vi "Set Hover.vi"(8 "error in (no error)":errorcluster, 9 "Set Hover (F)":bool, 10 "Index":i32, 11 "MCListbox with Checkboxes in":refnum<class "MCListbox with Checkboxes.lvclass">) -> (0 "error out":errorcluster, 3 "MCListbox with Checkboxes out":refnum<class "MCListbox with Checkboxes.lvclass">)   [LabVIEW 2016, in "MCListbox with Checkboxes.lvclass"]
uses:
  MCListbox with Checkboxes.lvclass
  MCListbox with Checkboxes.lvclass/MCListbox with Checkboxes.ctl
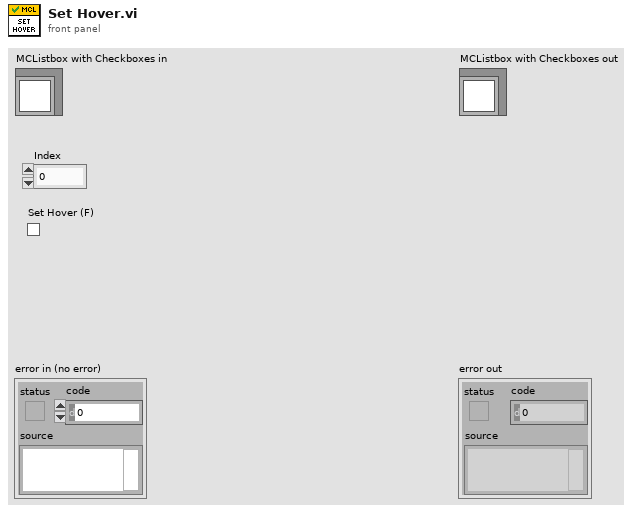
[diagram p1: front panel]
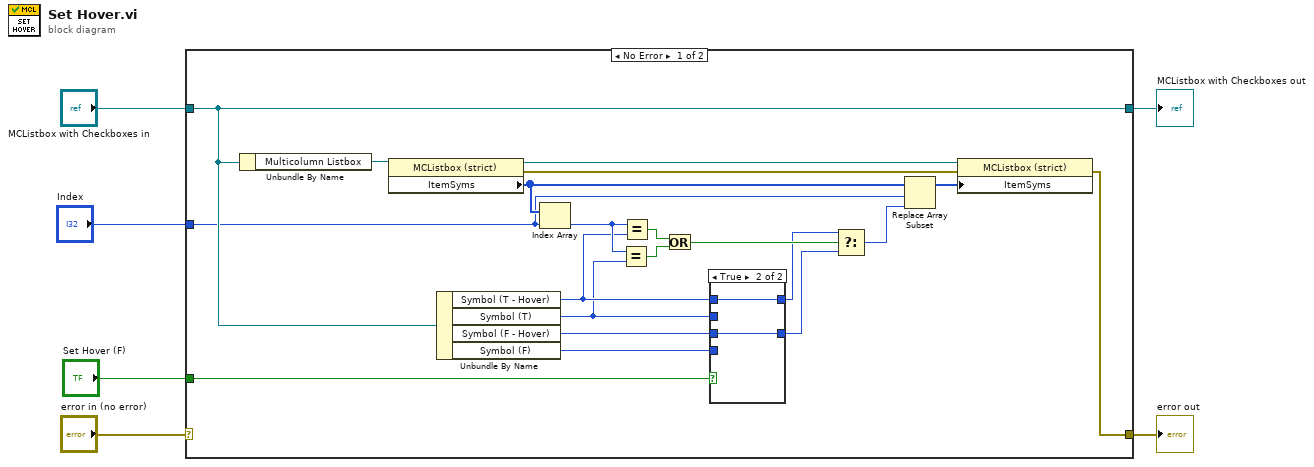
[diagram p0: block diagram]
diagram:
  n1 = case shown="No Error" "error in (no error)" {
    selector: "error in (no error)" -> [_ w32]
    tunnel: [w11 w32] -> w5
    tunnel: [w25 w31] -> w3
    tunnel: "MCListbox with Checkboxes in" -> [w25 w31]
    tunnel: "Index" -> [w8 _]
    tunnel: "Set Hover (F)" -> [w17 _]
    frame No Error {
      n2 = Unbundle By Name(w25) -> ("Multicolumn Listbox"=w26:refnum<vi>)
      n3 = property class="MCListbox (strict)"(reference=w26) -> (reference out=w13:refnum<vi>, error out=w12:errorcluster, "ItemSyms"=w9:i32[])  [unwired: 1 in]
      n4 = Unbundle By Name(w25) -> ("Symbol (T - Hover)"=w21:i32, "Symbol (T)"=w20:i32, "Symbol (F - Hover)"=w19:i32, "Symbol (F)"=w18:i32)
      n5 = Index Array(array=w9, index=w8) -> (element=w24:i32)
      n6 = Equal?(x=w24, y=w20) -> (x = y?=w22:bool)
      n7 = Equal?(x=w24, y=w21) -> (x = y?=w23:bool)
      n8 = Or(x=w23, y=w22) -> (x .or. y?=w16:bool)
      n9 = case shown="True" w17 {
        tunnel: w21 -> [_ w30]
        tunnel: w20 -> [w28 _]
        tunnel: w19 -> [_ w29]
        tunnel: w18 -> [w27 _]
        tunnel: [w28 w30] -> w15
        tunnel: [w27 w29] -> w14
        frame False {
        }
        frame True {
        }
      }
      n10 = Select(t=w15, s=w16, f=w14) -> (s? t:f=w7:i32)
      n11 = Replace Array Subset(array=w9, new element=w7, index=w8) -> (w10:i32[])
      n12 = property class="MCListbox (strict)"(reference=w13, error in=w12, "ItemSyms"=w10) -> (error out=w11:errorcluster)  [unwired: 1 out]
    }
    frame Error {
    }
  }
  "error out" <- w5
  "MCListbox with Checkboxes out" <- w3
